vi "Bin Indicator Control.vi"(0 "Bin Indicator Refs":T1[](array[typedef]), 1 "Init (F)":bool, 5 "Bin Levels":u16[](array[numeric])) -> ()   [LabVIEW 2020]
uses:
  Type Defs/Bin Indicator Type Def.ctl
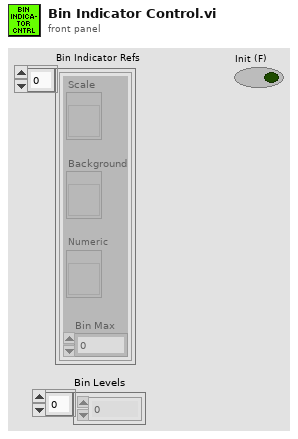
[diagram p1: front panel]
types:
  T1 = typedef "Bin Indicator Type Def.ctl" = cluster{"Scale":refnum<vi>, "Background":refnum<vi>, "Numeric":refnum<vi>, "Bin Max":u16}
  T2 = typedef "LVPositionTypeDef.ctl" = cluster{"Left":i32, "Top":i32}
  T3 = typedef "LVBoundsTypeDef.ctl" = cluster{"Width":u32, "Height":u32}
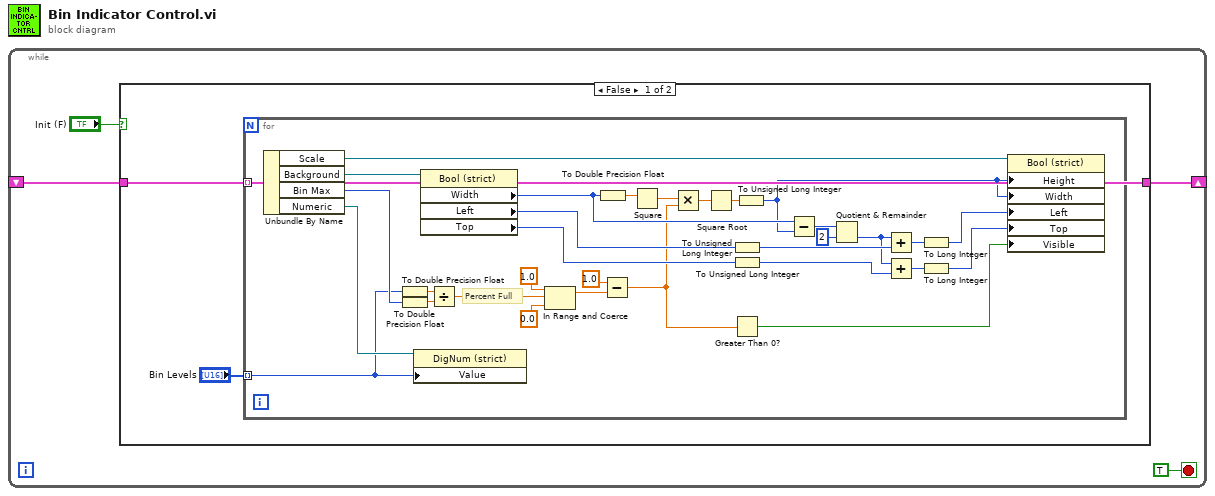
[diagram p0: block diagram]
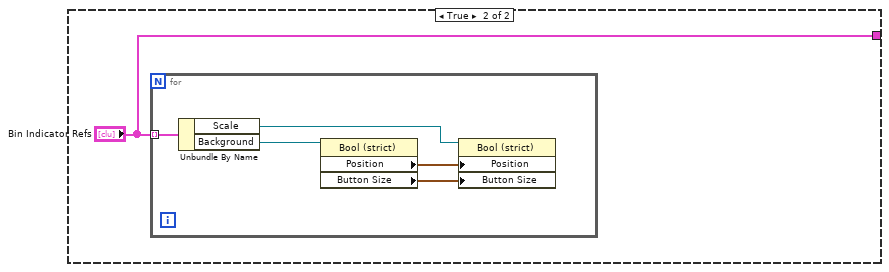
[diagram p2: hidden frame]
diagram:
  n1 = while {
    shift-right: [w2] -> _
    shift-left: _ -> [w1]
    stop <- TRUE stop-if-true
    n2 = case shown="False" "Init (F)" {
      tunnel: w1 -> [w6 _]
      tunnel: [w6 "Bin Indicator Refs"] -> w2
      frame False {
        n3 = for {
          tunnel: w6 -> [w38] mode=indexing
          tunnel: "Bin Levels" -> [w7] mode=indexing
          # "Percent Full"
          n4 = Unbundle By Name(w38) -> ("Scale"=w32:refnum<vi>, "Background"=w36:refnum<vi>, "Bin Max"=w35:u16, "Numeric"=w37:refnum<vi>)
          n5 = To Double Precision Float(number=w7) -> (double precision float=w34:dbl)
          n6 = To Double Precision Float(number=w35) -> (double precision float=w33:dbl)
          n7 = property class="DigNum (strict)"(reference=w37, "Value"=w7) -> ()  [unwired: 1 in, 2 out]
          n8 = property class="Bool (strict)"(reference=w36) -> ("Width"=w28:u32, "Left"=w24:i32, "Top"=w22:i32)  [unwired: 1 in, 2 out]
          n9 = Divide(x=w34, y=w33) -> (x/y=w31:dbl)
          n10 = In Range and Coerce(upper limit=1.0, x=w31, lower limit=0.0 ("upper limit")) -> (coerced(x)=w10:dbl)  [unwired: 1 out]
          n11 = To Double Precision Float(number=w28) -> (double precision float=w14:dbl)
          n12 = Subtract(x=1.0 ("upper limit"), y=w10) -> (x-y=w8:dbl)
          n13 = Square(x=w14) -> (x^2=w13:dbl)
          n14 = Multiply(x=w13, y=w8) -> (x*y=w12:dbl)
          n15 = Square Root(x=w12) -> (sqrt(x)=w11:dbl)
          n16 = To Unsigned Long Integer(number=w24) -> (unsigned 32bit integer=w23:u32)
          n17 = To Unsigned Long Integer(number=w22) -> (unsigned 32bit integer=w20:u32)
          n18 = Greater Than 0?(x=w8) -> (x > 0?=w9:bool)
          n19 = To Unsigned Long Integer(number=w11) -> (unsigned 32bit integer=w27:u32)
          n20 = Subtract(x=w28, y=w27) -> (x-y=w26:u32)
          n21 = Quotient & Remainder(x=w26, y=u32 2) -> (floor(x/y)=w21:u32)  [unwired: 1 out]
          n22 = Add(x=w21, y=w23) -> (x+y=w19:u32)
          n23 = Add(x=w21, y=w20) -> (x+y=w18:u32)
          n24 = To Long Integer(number=w19) -> (32bit integer=w17:i32)
          n25 = To Long Integer(number=w18) -> (32bit integer=w16:i32)
          n26 = property class="Bool (strict)"(reference=w32, "Height"=w27, "Width"=w27, "Left"=w17, "Top"=w16, "Visible"=w9) -> ()  [unwired: 1 in, 2 out]
        }
      }
      frame True {
        n27 = for {
          tunnel: "Bin Indicator Refs" -> [w40] mode=indexing
          n28 = Unbundle By Name(w40) -> ("Scale"=w42:refnum<vi>, "Background"=w41:refnum<vi>)
          n29 = property class="Bool (strict)"(reference=w41) -> ("Position"=w43:T2, "Button Size"=w44:T3)  [unwired: 1 in, 2 out]
          n30 = property class="Bool (strict)"(reference=w42, "Position"=w43, "Button Size"=w44) -> ()  [unwired: 1 in, 2 out]
        }
      }
    }
  }
